vi "relativ_path_to_absolute_path.vi"(11 "relativ path":path) -> (3 "absolute path":path)   [LabVIEW 2017]
doc: "Convert the application relativ path to an absolute path"
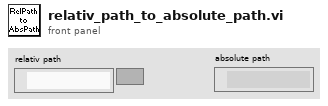
[diagram p1: front panel]
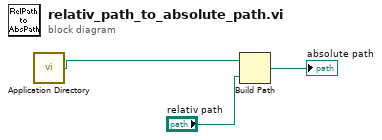
[diagram p0: block diagram]
diagram:
  n1 = call <vilib>:"Application Directory.vi"() -> ("Application Directory"=w1:path)
  n2 = Build Path(base path=w1, name or relative path="relativ path") -> (appended path=→"absolute path":path)
